vi "write tag name.vi"(8 "error in":errorcluster, 10 "name":string, 11 "system tag in":refnum<class "tag descriptor.lvclass">) -> (0 "error out":errorcluster, 3 "system tag out":refnum<class "tag descriptor.lvclass">)   [LabVIEW 2013, in "tag bus.lvlib" / "tag descriptor.lvclass"]
doc: "Writes the name of the tag, as stored in the tag descriptor."
uses:
  tag descriptor.lvclass
  tag descriptor.lvclass/tag descriptor.ctl
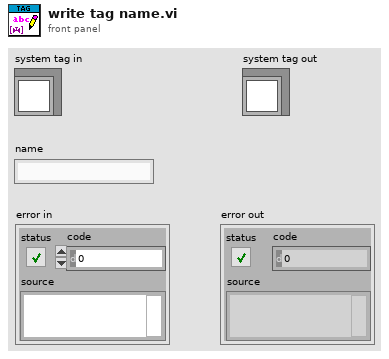
[diagram p1: front panel]
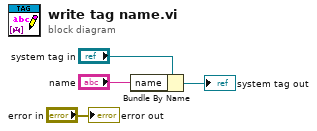
[diagram p0: block diagram]
diagram:
  n1 = Bundle By Name(cluster="system tag in", "name"="name") -> (→"system tag out":refnum<class "tag descriptor.lvclass">)
  "error out" <- "error in"
